vi "Teleop.vi"(10 "Match Info":T1={"Autonomous Elapsed Seconds"=0.0, "TeleOp Elapsed Seconds"=0.0, "Disabled Elapsed Seconds"=0.0, "Visited Autonomous"=FALSE, "Visited TeleOp"=FALSE, "Visited Disabled"=FALSE, "Autonomous Settings"={"Autonomous Style"=enum."Independent", "VI Refnum"=refnum}}, 11 "Call Context":T2) -> ()   [LabVIEW 2015]
doc: "This VI is called for each TeleOp packet received from the DS where the robot is not disabled. It is often used to read from the joysticks and update I/O or to update setpoints for timed control loops. It should complete and return within 20 milliseconds or it may miss DS packets."
uses:
  <vilib>/Rock Robotics/WPI/DriverStation/WPI_DriverStationDerivedRobotMode.ctl
  <vilib>/Rock Robotics/WPI/DriverStation/WPI_DriverStationMatch Info.ctl
  <vilib>/Rock Robotics/WPI/Solenoid/WPI_SolenoidValue.ctl
  <vilib>/Rock Robotics/WPI/Utilities/WPI_GetSetVariantRefNum.vi
  <vilib>/Rock Robotics/Network Tables/NT Read Boolean.vi
  <vilib>/Rock Robotics/Network Tables/NT Read Number.vi
  <vilib>/Rock Robotics/WPI/Solenoid/WPI_SolenoidSetEnum.vi
  <vilib>/addons/control/pid/pid.llb/PID (DBL).vi
  <vilib>/addons/control/pid/NI_PID_pid.lvlib
panel:
  out "Encodeur gauche max":dbl
  out "Encodeur droit max":dbl
  out "Encodeur gauche min":dbl
  out "Encodeur droit min":dbl
  out "Sample Slider 0":dbl(slide) scale=0.0..5.0
  out "Sample Boolean 1":bool
  out "Sample Boolean 0":bool
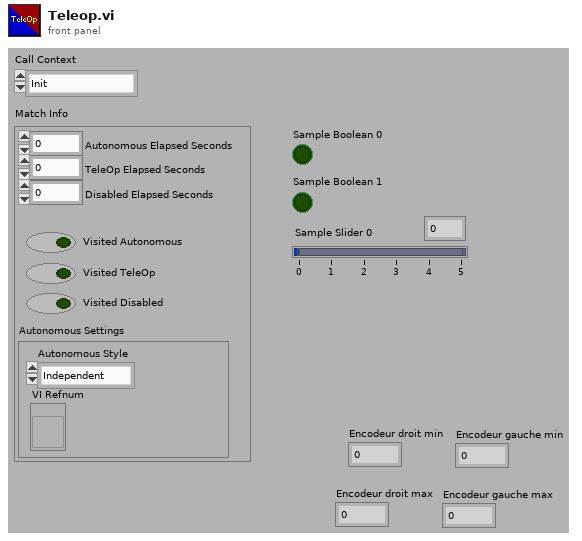
[diagram p1: front panel]
types:
  T1 = typedef "WPI_DriverStationMatch Info.ctl" = cluster{"Autonomous Elapsed Seconds":dbl, "TeleOp Elapsed Seconds":dbl, "Disabled Elapsed Seconds":dbl, "Visited Autonomous":bool, "Visited TeleOp":bool, "Visited Disabled":bool, "Autonomous Settings":cluster{"Autonomous Style":enum16{"Iterative", "Independent"}, "VI Refnum":refnum<vi>}}
  T2 = typedef "WPI_DriverStationDerivedRobotMode.ctl" = enum16{"Init", "Execute", "Stop"}
  T3 = typedef "WPI_SolenoidValue.ctl" = enum16{"Off", "On", "Forward", "Reverse"}
  T4 = typedef "WPI_SolenoidDevRef.ctl" = cluster{"DevStatus":errorcluster, "Pneumatics Control Module":u8, "Forward Solenoid Channel":T5, "Reverse Solenoid Channel":T5}
  T5 = typedef "WPI_SolenoidChannel.ctl" = enum8{"Solenoid 0", "Solenoid 1", "Solenoid 2", "Solenoid 3", "Solenoid 4", "Solenoid 5", "Solenoid 6", "Solenoid 7", "Invalid"}
  T6 = typedef "WPI_JoystickDevRef.ctl" = cluster{"Device":T7}
  T7 = typedef "WPI_JoystickDeviceEnum.ctl" = enum16{"USB 0", "USB 1", "USB 2", "USB 3", "USB 4", "USB 5"}
  T8 = cluster{"Buttons[0]":bool, "Buttons[1]":bool, "Buttons[2]":bool, "Buttons[3]":bool, "Buttons[4]":bool, "Buttons[5]":bool, "Buttons[6]":bool, "Buttons[7]":bool, "Buttons[8]":bool}
  T9 = cluster{"Axes[0]":dbl, "Axes[1]":dbl, "Axes[2]":dbl, "Axes[3]":dbl, "Axes[4]":dbl, "Axes[5]":dbl, "Axes[6]":dbl, "Axes[7]":dbl, "Axes[8]":dbl}
  T10 = typedef "WPI_ServoDeviceRef.ctl" = cluster{"DeviceStatus":errorcluster, "PWM Channel":T11, "DeadBand":T12}
  T11 = typedef "FPGA_DIOPWMChannel.ctl" = enum8{"PWM 0", "PWM 1", "PWM 2", "PWM 3", "PWM 4", "PWM 5", "PWM 6", "PWM 7", "PWM 8", "PWM 9", "PWM MXP 0", "PWM MXP 1", "PWM MXP 2", "PWM MXP 3", "PWM MXP 4", "PWM MXP 5", "PWM MXP 6", "PWM MXP 7", "PWM MXP 8", "PWM MXP 9", "Invalid"}
  T12 = typedef "WPI_PWMDeadband.ctl" = cluster{"Name":string, "maxPositivePwm":i32, "minPositivePwm":i32, "centerPwm":i32, "maxNegativePwm":i32, "minNegativePwm":i32, "angularRange":u16}
  T13 = typedef "WPI_EncoderDevRef.ctl" = cluster{"DevStatus":errorcluster, "EncoderIndex":T14, "CounterIndex":T15, "DistancePerCount":dbl, "Decoding Type":T16}
  T14 = typedef "FPGA_EncoderIdx.ctl" = enum8{"Enc 0", "Enc 1", "Enc 2", "Enc 3", "Enc 4", "Enc 5", "Enc 6", "Enc 7", "Invalid"}
  T15 = typedef "FPGA_CounterCtrSystemIndex.ctl" = enum8{"Ctr 0", "Ctr 1", "Ctr 2", "Ctr 3", "Ctr 4", "Ctr 5", "Ctr 6", "Ctr 7", "Invalid"}
  T16 = typedef "WPI_EncoderType.ctl" = enum16{"1x", "2x", "4x"}
  T17 = cluster{"proportional gain (Kc)":dbl, "integral time (Ti, min)":dbl, "derivative time (Td, min)":dbl}
  T18 = typedef "WPI_MotorControlDeviceRef.ctl" = cluster{"DeviceStatus":errorcluster, "Type":T19, "PWM":cluster{"PWM Channel":T11, "DeadBand":T12}, "CAN":cluster{"Device Number":u8, "Control Mode":T20, "Semaphore":T21, "Max Vout":dbl, "TalonSRX Control Mode":T22}, "Invert":bool}
  T19 = typedef "WPI_MotorControlType.ctl" = enum16{"PWM", "CAN", "CANTalonSRX"}
  T20 = typedef "WPI_CANJaguar_ControlMode.ctl" = enum8{"Percent VBus", "Current", "Speed", "Position", "Voltage"}
  T21 = typedef "Semaphore RefNum" = refnum<k1>
  T22 = typedef "WPI_CANTalonSRX_APIControlMode.ctl" = enum8{"Percent VBus", "Speed", "Position", "Slave", "Unchanged / Invalid", "Voltage Compensation", "Current", "Motion Profile"}
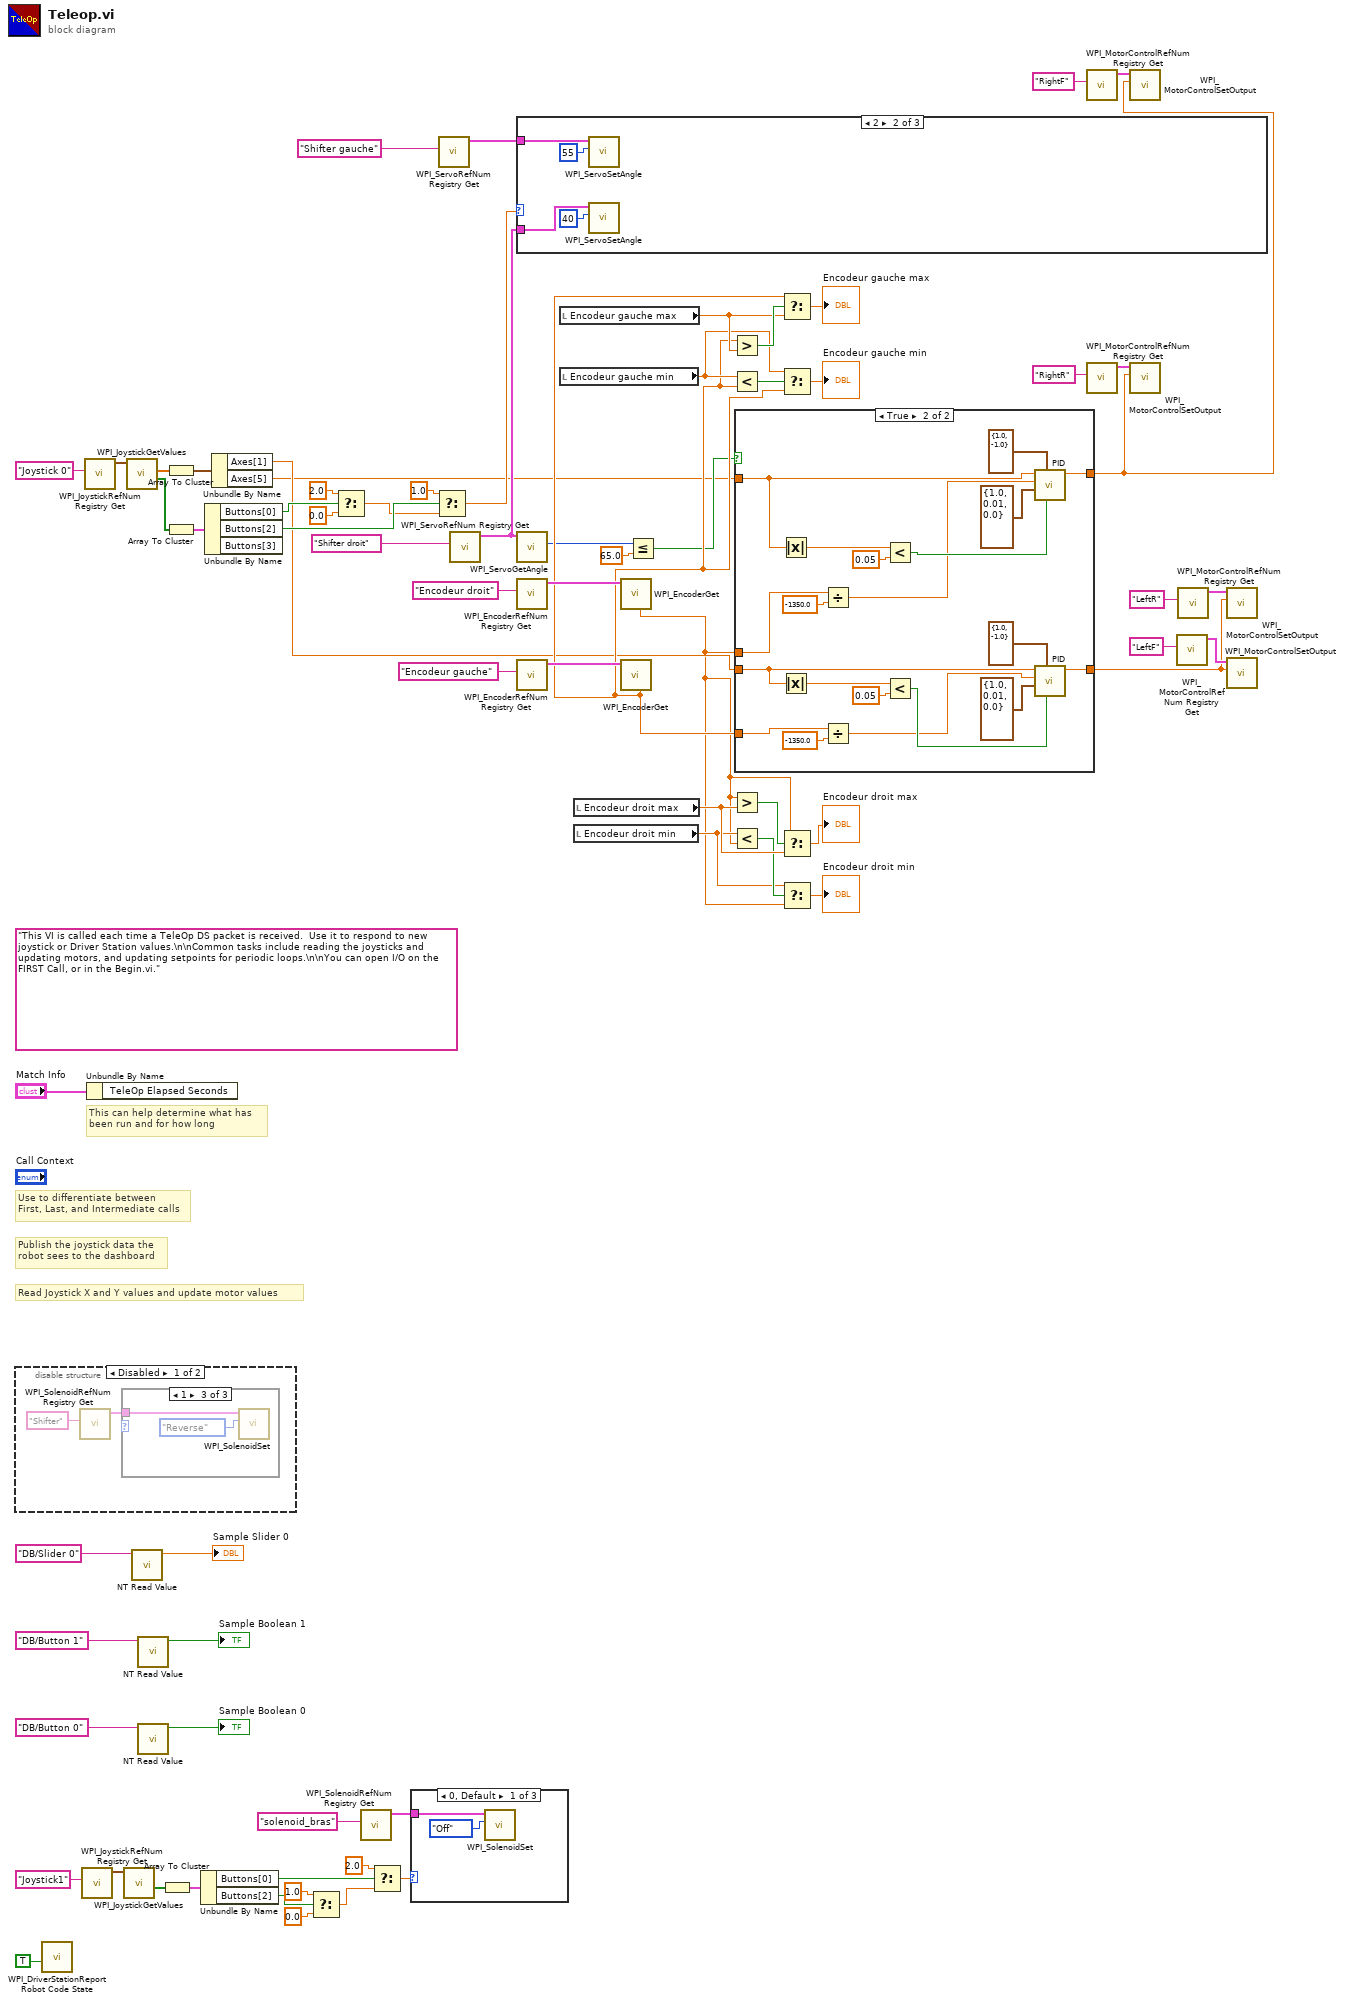
[diagram p0: block diagram]
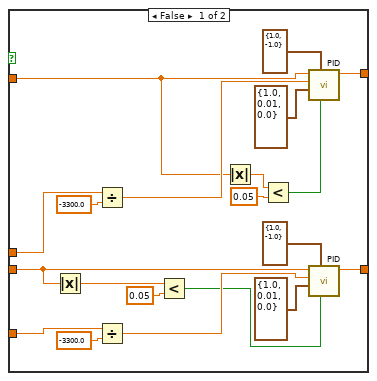
[diagram p2: hidden frame]
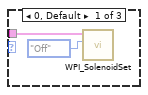
[diagram p3: hidden frame]
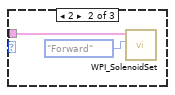
[diagram p4: hidden frame]
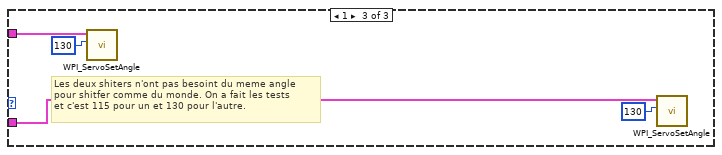
[diagram p7: hidden frame]
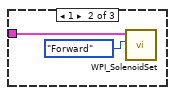
[diagram p8: hidden frame]
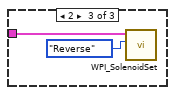
[diagram p9: hidden frame]
diagram:
  (unwired) "This VI is called each time a TeleOp DS packet is received.  Use it to respond to new joystick or Driver Station values.\n\nCommon tasks include reading the joysticks and updating motors, and updating setpoints for periodic loops.\n\nYou can open I/O on the FIRST Call, or in the Begin.vi."
  # "Publish the joystick data the\nrobot sees to the dashboard"
  # "Use to differentiate between\nFirst, Last, and Intermediate calls"
  # "This can help determine what has\nbeen run and for how long"
  # "Read Joystick X and Y values and update motor values"
  n1 = disable-structure shown="Disabled" {
    frame Disabled {
      n2 = call <vilib>:"WPI_SolenoidRefNum Registry Get.vi"("refnum name"="Shifter") -> ("SolenoidDevRef"=w73:T4)  [unwired: 9 in, 1 out]
      n3 = case shown="1" {
        selector: _ -> [_ _ _]
        tunnel: w73 -> [w75 w77 w78]
        frame 0, Default {
          n4 = call-poly <vilib>:"WPI_SolenoidSet.vi"("Value"=WPI_SolenoidValue."Off", "SolenoidDevRef"=w75) -> ()  [unwired: 8 in, 2 out]
        }
        frame 2 {
          n5 = call-poly <vilib>:"WPI_SolenoidSet.vi"("Value"=WPI_SolenoidValue."Forward", "SolenoidDevRef"=w77) -> ()  [unwired: 8 in, 2 out]
        }
        frame 1 {
          n6 = call-poly <vilib>:"WPI_SolenoidSet.vi"("Value"=WPI_SolenoidValue."Reverse", "SolenoidDevRef"=w78) -> ()  [unwired: 8 in, 2 out]
        }
      }
    }
    frame Enabled {
    }
  }
  n7 = call <vilib>:"WPI_DriverStationReport Robot Code State.vi"("TeleOp"=TRUE ("Autonomous")) -> ()  [unwired: 10 in, 1 out]
  n8 = call <vilib>:"WPI_JoystickRefNum Registry Get.vi"("refnum name"="Joystick1") -> ("JoystickDevRef"=w50:T6)  [unwired: 1 in, 9 out]
  n9 = call <vilib>:"WPI_JoystickRefNum Registry Get.vi"("refnum name"="Joystick 0") -> ("JoystickDevRef"=w69:T6)  [unwired: 1 in, 9 out]
  n10 = Unbundle By Name("Match Info") -> ()  [unwired: 1 out]
  n11 = call <vilib>:"WPI_JoystickGetValues.vi"("JoystickDevRef"=w50) -> ("Buttons"=w51:bool[])  [unwired: 6 in, 4 out]
  n12 = call <vilib>:"WPI_JoystickGetValues.vi"("JoystickDevRef"=w69) -> ("Buttons"=w61:bool[], "Axes"=w63:dbl[])  [unwired: 6 in, 3 out]
  n13 = call-poly <vilib>:"NT Read Value.vi"("Name"="DB/Slider 0" ("refnum name")) -> ("Numeric"=→"Sample Slider 0":dbl)  [unwired: 9 in, 1 out]
  n14 = call-poly <vilib>:"NT Read Value.vi"("Name"="DB/Button 1" ("refnum name")) -> ("Boolean"=→"Sample Boolean 1":bool)  [unwired: 9 in, 1 out]
  n15 = call-poly <vilib>:"NT Read Value.vi"("Name"="DB/Button 0" ("refnum name")) -> ("Boolean"=→"Sample Boolean 0":bool)  [unwired: 9 in, 1 out]
  n16 = Array To Cluster(array=w51) -> (cluster=w52:T8)
  n17 = Array To Cluster(array=w63) -> (cluster=w62:T9)
  n18 = Array To Cluster(array=w61) -> (cluster=w60:T8)
  n19 = Unbundle By Name(w52) -> ("Buttons[0]"=w45:bool, "Buttons[2]"=w44:bool)
  n20 = Unbundle By Name(w60) -> ("Buttons[0]"=w59:bool, "Buttons[2]"=w56:bool)  [unwired: 1 out]
  n21 = Unbundle By Name(w62) -> ("Axes[1]"=w8:dbl, "Axes[5]"=w3:dbl)
  n22 = Select(t=1.0, s=w44, f=0.0) -> (s? t:f=w46:dbl)
  n23 = Select(t=2.0, s=w59, f=0.0) -> (s? t:f=w55:dbl)
  n24 = call <vilib>:"WPI_SolenoidRefNum Registry Get.vi"("refnum name"="solenoid_bras") -> ("SolenoidDevRef"=w39:T4)  [unwired: 9 in, 1 out]
  n25 = Select(t=2.0, s=w45, f=w46) -> (s? t:f=w40:dbl)
  n26 = case shown="0, Default" w40 {
    tunnel: w39 -> [w80 w83 w84]
    frame 0, Default {
      n27 = call-poly <vilib>:"WPI_SolenoidSet.vi"("Value"=WPI_SolenoidValue."Off", "SolenoidDevRef"=w80) -> ()  [unwired: 8 in, 2 out]
    }
    frame 1 {
      n28 = call-poly <vilib>:"WPI_SolenoidSet.vi"("Value"=WPI_SolenoidValue."Forward", "SolenoidDevRef"=w83) -> ()  [unwired: 8 in, 2 out]
    }
    frame 2 {
      n29 = call-poly <vilib>:"WPI_SolenoidSet.vi"("Value"=WPI_SolenoidValue."Reverse", "SolenoidDevRef"=w84) -> ()  [unwired: 8 in, 2 out]
    }
  }
  n30 = Select(t=1.0, s=w56, f=w55) -> (s? t:f=w35:dbl)
  n31 = call <vilib>:"WPI_ServoRefNum Registry Get.vi"("refnum name"="Shifter gauche") -> ("ServoDeviceRef"=w36:T10)  [unwired: 9 in, 1 out]
  n32 = call <vilib>:"WPI_ServoRefNum Registry Get.vi"("refnum name"="Shifter droit") -> ("ServoDeviceRef"=w7:T10)  [unwired: 9 in, 1 out]
  n33 = case shown="2" w35 {
    tunnel: w36 -> [_ w89 w93]
    tunnel: w7 -> [_ w88 w92]
    frame 0, Default {
    }
    frame 2 {
      n34 = call <vilib>:"WPI_ServoSetAngle.vi"("Angle"=55, "ServoDeviceRef"=w89) -> ()  [unwired: 8 in, 2 out]
      n35 = call <vilib>:"WPI_ServoSetAngle.vi"("Angle"=40, "ServoDeviceRef"=w88) -> ()  [unwired: 8 in, 2 out]
    }
    frame 1 {
      # "Les deux shiters n'ont pas besoint du meme angle \npour shitfer comme du monde. On a fait les tests \net c'est 115 pour un et 130 pour l'autre."
      n36 = call <vilib>:"WPI_ServoSetAngle.vi"("Angle"=130, "ServoDeviceRef"=w93) -> ()  [unwired: 8 in, 2 out]
      n37 = call <vilib>:"WPI_ServoSetAngle.vi"("Angle"=130, "ServoDeviceRef"=w92) -> ()  [unwired: 8 in, 2 out]
    }
  }
  n38 = call <vilib>:"WPI_ServoGetAngle.vi"("ServoDeviceRef"=w7) -> ("Angle"=w5:u16)  [unwired: 7 in, 2 out]
  n39 = call <vilib>:"WPI_EncoderRefNum Registry Get.vi"("refnum name"="Encodeur droit") -> ("EncoderDevRef"=w33:T13)  [unwired: 9 in, 1 out]
  n40 = call <vilib>:"WPI_EncoderRefNum Registry Get.vi"("refnum name"="Encodeur gauche") -> ("EncoderDevRef"=w32:T13)  [unwired: 9 in, 1 out]
  n41 = local read "Encodeur gauche max"() -> (w29:dbl)
  n42 = local read "Encodeur gauche min"() -> (w26:dbl)
  n43 = local read "Encodeur droit max"() -> (w23:dbl)
  n44 = local read "Encodeur droit min"() -> (w21:dbl)
  n45 = call <vilib>:"WPI_EncoderGet.vi"("EncoderDevRef"=w33) -> ("Rate"=w2:dbl)  [unwired: 5 in, 5 out]
  n46 = call <vilib>:"WPI_EncoderGet.vi"("EncoderDevRef"=w32) -> ("Rate"=w10:dbl)  [unwired: 5 in, 5 out]
  n47 = Less Or Equal?(x=w5, y=65.0) -> (x <= y?=w4:bool)
  n48 = Greater?(x=w10, y=w29) -> (0:w30:bool)
  n49 = Less?(x=w26, y=w10) -> (x < y?=w27:bool)
  n50 = Greater?(x=w2, y=w23) -> (0:w24:bool)
  n51 = Less?(x=w21, y=w2) -> (x < y?=w22:bool)
  n52 = case shown="True" w4 {
    tunnel: w10 -> [w97 w125]
    tunnel: w8 -> [w95 w124]
    tunnel: [w99 w126] -> w9
    tunnel: w3 -> [w94 w114]
    tunnel: w2 -> [w96 w116]
    tunnel: [w98 w115] -> w1
    frame False {
      n53 = Absolute Value(x=w95) -> (abs(x)=w112:dbl)
      n54 = Divide(x=w96, y=-3300.0) -> (x/y=w103:dbl)
      n55 = Divide(x=w97, y=-3300.0) -> (x/y=w110:dbl)
      n56 = Less?(x=w112, y=0.05) -> (x < y?=w100:bool)
      n57 = Absolute Value(x=w94) -> (abs(x)=w105:dbl)
      n58 = Less?(x=w105, y=0.05) -> (x < y?=w107:bool)
      n59 = call-poly <vilib>:"PID.vi"("reinitialize? (F)"=w107, "output range"=cluster{"output high":dbl, "output low":dbl} {"output high"=1.0, "output low"=-1.0}, "PID gains"=T17 {"proportional gain (Kc)"=1.0, "integral time (Ti, min)"=0.01, "derivative time (Td, min)"=0.0}, "process variable"=w103, "setpoint"=w94) -> ("output"=w98:dbl)  [unwired: 5 in, 1 out]
      n60 = call-poly <vilib>:"PID.vi"("reinitialize? (F)"=w100, "output range"=cluster{"output high":dbl, "output low":dbl} {"output high"=1.0, "output low"=-1.0}, "PID gains"=T17 {"proportional gain (Kc)"=1.0, "integral time (Ti, min)"=0.01, "derivative time (Td, min)"=0.0}, "process variable"=w110, "setpoint"=w95) -> ("output"=w99:dbl)  [unwired: 5 in, 1 out]
    }
    frame True {
      n61 = Absolute Value(x=w114) -> (abs(x)=w121:dbl)
      n62 = Absolute Value(x=w124) -> (abs(x)=w131:dbl)
      n63 = Divide(x=w116, y=-1350.0) -> (x/y=w119:dbl)
      n64 = Divide(x=w125, y=-1350.0) -> (x/y=w129:dbl)
      n65 = Less?(x=w121, y=0.05) -> (x < y?=w123:bool)
      n66 = Less?(x=w131, y=0.05) -> (x < y?=w133:bool)
      n67 = call-poly <vilib>:"PID.vi"("reinitialize? (F)"=w123, "output range"=cluster{"output high":dbl, "output low":dbl} {"output high"=1.0, "output low"=-1.0}, "PID gains"=T17 {"proportional gain (Kc)"=1.0, "integral time (Ti, min)"=0.01, "derivative time (Td, min)"=0.0}, "process variable"=w119, "setpoint"=w114) -> ("output"=w115:dbl)  [unwired: 5 in, 1 out]
      n68 = call-poly <vilib>:"PID.vi"("reinitialize? (F)"=w133, "output range"=cluster{"output high":dbl, "output low":dbl} {"output high"=1.0, "output low"=-1.0}, "PID gains"=T17 {"proportional gain (Kc)"=1.0, "integral time (Ti, min)"=0.01, "derivative time (Td, min)"=0.0}, "process variable"=w129, "setpoint"=w124) -> ("output"=w126:dbl)  [unwired: 5 in, 1 out]
    }
  }
  n69 = Select(t=w10, s=w30, f=w29) -> (s? t:f=→"Encodeur gauche max":dbl)
  n70 = Select(t=w26, s=w27, f=w10) -> (s? t:f=→"Encodeur gauche min":dbl)
  n71 = Select(t=w2, s=w24, f=w23) -> (s? t:f=→"Encodeur droit max":dbl)
  n72 = Select(t=w21, s=w22, f=w2) -> (s? t:f=→"Encodeur droit min":dbl)
  n73 = call <vilib>:"WPI_MotorControlRefNum Registry Get.vi"("refnum name"="RightF") -> ("MotorControlDevRef"=w16:T18)  [unwired: 9 in, 1 out]
  n74 = call <vilib>:"WPI_MotorControlRefNum Registry Get.vi"("refnum name"="RightR") -> ("MotorControlDevRef"=w15:T18)  [unwired: 9 in, 1 out]
  n75 = call <vilib>:"WPI_MotorControlSetOutput.vi"("Output"=w1, "MotorControlDevRef"=w16) -> ()  [unwired: 7 in, 3 out]
  n76 = call <vilib>:"WPI_MotorControlSetOutput.vi"("Output"=w1, "MotorControlDevRef"=w15) -> ()  [unwired: 7 in, 3 out]
  n77 = call <vilib>:"WPI_MotorControlRefNum Registry Get.vi"("refnum name"="LeftF") -> ("MotorControlDevRef"=w18:T18)  [unwired: 9 in, 1 out]
  n78 = call <vilib>:"WPI_MotorControlRefNum Registry Get.vi"("refnum name"="LeftR") -> ("MotorControlDevRef"=w17:T18)  [unwired: 9 in, 1 out]
  n79 = call <vilib>:"WPI_MotorControlSetOutput.vi"("Output"=w9, "MotorControlDevRef"=w17) -> ()  [unwired: 7 in, 3 out]
  n80 = call <vilib>:"WPI_MotorControlSetOutput.vi"("Output"=w9, "MotorControlDevRef"=w18) -> ()  [unwired: 7 in, 3 out]
